vi "DI Counter Sim Data.vi"(10 "DI Counter in":u32) -> (2 "DI Counter out":u32)   [LabVIEW 2014, in "SimSyA.lvlib"]
uses:
  SimSyA.lvlib
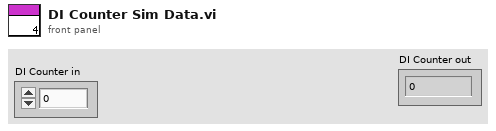
[diagram p1: front panel]
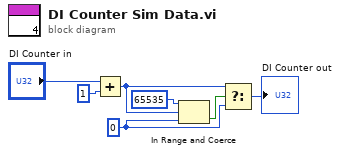
[diagram p0: block diagram]
diagram:
  w2 = u32 0 ("lower limit")
  n1 = Add(x="DI Counter in", y=u32 1) -> (x+y=w3:u32)
  n2 = In Range and Coerce(upper limit=u32 65535, x=w3, lower limit=w2) -> (In Range?=w4:bool)  [unwired: 1 out]
  n3 = Select(t=w3, s=w4, f=w2) -> (s? t:f=→"DI Counter out":u32)
